vi "osa_parse init result.vi"(8 "wipe content?":bool, 10 "serial response in":string, 11 "OSB status/control refnum in":refnum<vi>) -> ()   [LabVIEW 2021]
panel:
  # "OSA subVI: parse init result and update main panel display"
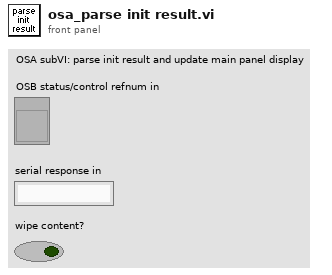
[diagram p1: front panel]
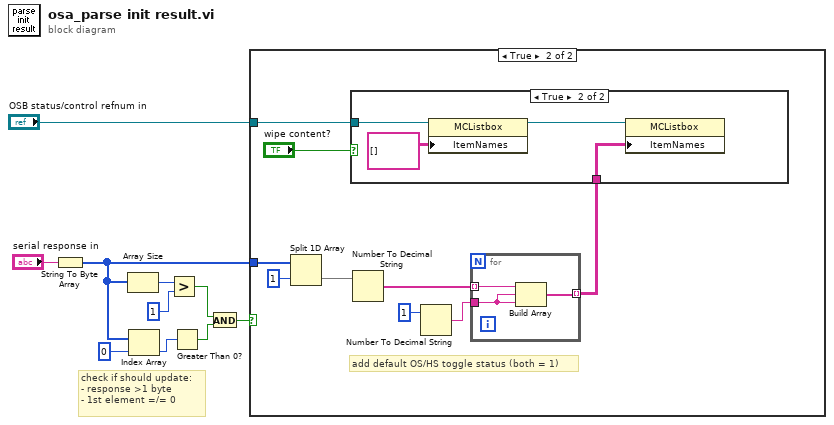
[diagram p0: block diagram]
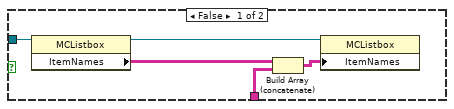
[diagram p3: hidden frame]
diagram:
  # "check if should update:\n- response >1 byte\n- 1st element =/= 0"
  n1 = String To Byte Array(string="serial response in") -> (unsigned byte array=w2:u8[])
  n2 = Array Size(array=w2) -> (size(s)=w5:i32)
  n3 = Index Array(array=w2, index=0) -> (element=w6:u8)
  n4 = Greater?(x=w5, y=1) -> (0:w7:bool)
  n5 = Greater Than 0?(x=w6) -> (x > 0?=w8:bool)
  n6 = And(x=w7, y=w8) -> (x .and. y?=w9:bool)
  n7 = case shown="True" w9 {
    tunnel: w2 -> [_ w18]
    tunnel: "OSB status/control refnum in" -> [_ w14]
    frame False {
    }
    frame True {
      # "add default OS/HS toggle status (both = 1)"
      n8 = Split 1D Array(array=w18, index=1) -> (second subarray=w15:u8[])  [unwired: 1 out]
      n9 = Number To Decimal String(number=w15) -> (decimal integer string=w16:string[])  [unwired: 1 in]
      n10 = Number To Decimal String(number=1) -> (decimal integer string=w13:string)  [unwired: 1 in]
      n11 = for {
        tunnel: w16 -> [w22] mode=indexing
        tunnel: w13 -> [w21]
        tunnel: [w20] -> w11 mode=indexing
        n12 = Build Array(w22, w21, w21) -> (w20:string[])
      }
      n13 = case shown="True" "wipe content?" {
        tunnel: w14 -> [w27 w30]
        tunnel: w11 -> [w23 w31]
        frame False {
          n14 = property class="MCListbox"(reference=w27) -> (reference out=w25:refnum<vi>, "ItemNames"=w26:string[][])  [unwired: 1 in, 1 out]
          n15 = Build Array (concatenate)(w26, w23) -> (w24:string[][])
          n16 = property class="MCListbox"(reference=w25, "ItemNames"=w24) -> ()  [unwired: 1 in, 2 out]
        }
        frame True {
          n17 = property class="MCListbox"(reference=w30, "ItemNames"=string[][] [] ("Item Names")) -> (reference out=w29:refnum<vi>)  [unwired: 1 in, 1 out]
          n18 = property class="MCListbox"(reference=w29, "ItemNames"=w31) -> ()  [unwired: 1 in, 2 out]
        }
      }
    }
  }
